vi "Get App Name and Dir.vi"(8 "错误输入":errorcluster) -> (0 "错误输出":errorcluster, 2 "AppDir":path, 3 "AppName":string)   [LabVIEW 2012, in "Application.lvlib"]
uses:
  Application.lvlib
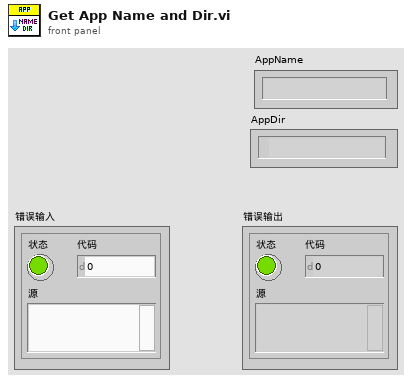
[diagram p1: front panel]
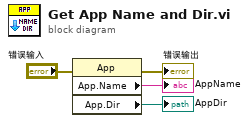
[diagram p0: block diagram]
diagram:
  n1 = property class="App"(error in="错误输入") -> (error out=→"错误输出":errorcluster, "App.Name"=→"AppName":string, "App.Dir"=→"AppDir":path)  [unwired: 1 in, 1 out]
